vi "Main_FPGA.vi"() -> ()   [LabVIEW 2021]
uses:
  <vilib>/Platform/TimedLoop/XDataNode/timing_clust.ctl
  <vilib>/Platform/TimedLoop/XDataNode/nitl_modes.ctl
  <vilib>/Platform/TimedLoop/XDataNode/wakeup.ctl
  <vilib>/rvi/Emulation/niFpgaGetClockAttributes.vi
  <vilib>/rvi/Emulation/niFpgaSctlEmulationGetInTimedLoop.vi
  <vilib>/rvi/Emulation/niFpgaEmulationReportErrorSimple.vi
  <vilib>/rvi/Emulation/niFpgaProcessEmulError.vi
  <vilib>/rvi/Emulation/niFpgaCriticalErrorInLSC.vi
  <vilib>/rvi/eio/common/nirviEmuTemplateMethod_errors.vi
  <vilib>/Platform/TimedLoop/XDataNode/XDataNode.xnode
  <vilib>/eio/EIONode/EIONode.xnode
  <vilib>/Platform/TimedLoop/XDataNode/XDNodeRunTimeDep.lvlib
panel:
  out "CH1 SS Time (200ns)":u32
  out "CH1 Stoping":bool
  out "CH1 3rd harmonic (kHz)":fxp<+,20,10> caption="Actual frequency (kHz)" format="%#.3f"
  in  "CH2":bool
  in  "CH1":bool caption="Hardware trigger\nin enable"
  in  "Output trigger \nfrequency (Hz)":u32=30 caption="Camera frequency (Hz)" min=1 max=200
  out "CH2 Trigger Tab":enum32{"Page 1", "Page 2"}(tab) caption="CH2 trigger"
  in  "CH2 trigger":bool
  out "CH2 trigger 2":bool=TRUE
  out "Ch1 Trigger Tab":enum32{"Page 1", "Page 2"}(tab) caption="CH1 trigger"
  in  "CH1 trigger":bool
  out "CH1 trigger 2":bool=TRUE
  out "Syn tab":enum32{"Page 1", "Page 2"}(tab) caption="Synchronous trigger"
  in  "Synchronous trigger 2":bool
  out "Syn Boolean 2":bool=TRUE
  out "CH2 cooling":bool
  out "CH2 Status":T1(tab) caption="Status:"
  out "CH1 cooling":bool
  out "CH1 Status":T1(tab) caption="Status:"
  in  "Tab Control 2":enum32{"Notes", "Others"}(tab)
  out "CH2 no cooling":u32
  out "CH2 delay (200ns)":u32
  out "CH2 pulse period (200ns)":u32
  out "CH2 ON":bool
  out "CH2 Total time (200ns)":u32
  out "CH2 On time (200ns)":u32
  out "CH2 duty ratio":u32
  out "CH2 step (Hz)":u32
  out "CH2 actual f (kHz)":fxp<+,20,10> caption="Board frequency (kHz)"
  in  "CH2 maximum absolute amp":fxp<+,32,1>=0.125 caption="Maximum duty ratio"
  out "CH2 T is longer than 14 mins":bool
  out "CH2 Total T1 is longer than 4s":bool
  in  "Tab Control 1":enum32{"Notes", "Others"}(tab)
  out "CH1 step (Hz)":u32
  out "CH1 duty ratio":u32
  out "CH1 on time (200ns)":u32
  out "CH1 Pulse period (200ns)":u32
  out "CH1 ON":bool
  out "N of 5MHz":i32
  out "CH1 Total time (200ns)":u32
  out "CH1 delay (200ns)":u32
  out "CH1 no cooling":u32
  in  "CH1 maximum absolute amp":fxp<+,32,1>=0.0400000000372529 caption="Maximum duty ratio"
  out "CH1 T too long":bool
  out "CH1 T1 too long":bool
  out "DIO0":bool
  out "CH1 actual f (kHz)":fxp<+,20,10> caption="Board frequency (kHz)" format="%#.3g"
  out "CH1 Starting":bool
  in  "CH1 SS slope":u32=3 caption="Slope (duty raio% / 10ms)" max=50
  out "CH1 soft SS?":bool
  out "CH1 SS time (sec)":fxp<+,16,0>=0.0009765625 caption="Soft start/stop time (s)" format="%#.4f"
  out "CH2 elapsed time (sec)":fxp<+,40,20> caption="Elapsed time (s)" format="%#.3f"
  out "CH2 status":bool=TRUE caption="Status"
  out "CH2 3rd harmonic (kHz)":fxp<+,20,10> caption="Actual frequency (kHz)" format="%#.3f"
  in  "CH2 frequency (kHz)":fxp<+,32,20>=543.0 caption="Frequency (kHz)" format="%#.1f"
  in  "CH2 T1 time (sec)":fxp<+,16,3>=0.0009765625 caption="T1 (s)" format="%#.3f"
  in  "CH2 T2 time (sec)":fxp<+,20,10>=0.0009765625 caption="T2 (s)" format="%#.3f"
  in  "CH2 normalized amp %":u8(slide)=62 caption="Normalized amp %" max=100 scale=0.0..100.0
  out "CH2 actual amp":fxp<+,32,7> caption="Duty ratio"
  in  "CH2 delay (sec)":fxp<+,20,10>=1.0 caption="Delay (s)" format="%#.3f"
  in  "Number of CH2 pulses":u8=1 caption="Pulses #" min=1 max=25
  out "CH2 Total time (sec)":fxp<+,32,20> caption="Total time (s)" format="%#.3f"
  out "CH2 cooling time (sec)":fxp<+,44,24>=3600.0 caption="Cooling time (s)" format="%#.3f"
  out "CH1 cooling time (sec)":fxp<+,44,24>=3600.0 caption="Cooling time (s)" format="%#.3f"
  out "CH1 Total time (sec)":fxp<+,32,20> caption="Total time (s)" format="%#.3f"
  out "CH1 status":bool=TRUE caption="Status"
  in  "CH1 delay (sec)":fxp<+,20,10>=1.0 caption="Delay (s)" format="%#.3f"
  in  "Number of CH1 pulses":u8=1 caption="Pulse #" min=1 max=25
  out "CH1 actual amp":fxp<+,32,7> caption="Duty ratio"
  in  "CH1 normalized amp %":u8(slide)=59 caption="Normalized amp %" max=100 scale=0.0..100.0
  in  "System on/off":bool
  out "CH1 elapsed time (sec)":fxp<+,40,20> caption="Elapsed time (s)" format="%#.3f"
  in  "CH1 T2 time (sec)":fxp<+,20,10>=0.0009765625 caption="T2 (s)" format="%#.3f"
  in  "CH1 T1 time (sec)":fxp<+,16,3>=0.0009765625 caption="T1 (s)" format="%#.3f"
  in  "CH1 frequency (kHz)":fxp<+,32,20>=48.89990234375 caption="Frequency (kHz)" format="%#.2f"
  # "! TURN ON !\n! CIRCULATION !\n! PUMP/CHILLER !"
  # "Channel 1: ~50kHz"
  # "Trigger"
  # "%"
  # "%"
  # "Channel 2: ~550kHz"
  # "Trigger"
  # "%"
  # "%"
  # "Idle"
  # "Running"
  # "Cooling"
  # "Error: \nTotal T1 is longer than 4 s"
  # "Error: \nTotal time is longer than 14 minutes"
  # "Idle"
  # "Running"
  # "Cooling"
  # "Error: \nTotal T1 is longer than 4 s"
  # "Error: \nTotal time is longer than 14 minutes"
  # "Notes\n\n1. 12% duty ratio is about 260A, which can produce about 12.5mT field.\n\n2. The total T1 cannot be longer than 4 seconds. After running, the system must wait 50 times of total T1 to cooling down.\n\n3. The total time = Delay time + Number of pulses * (T1+T2)+Cooling time, which cannot be longer than 14 minutes."
  # "Notes\n\n1. 4.1% duty ratio is about 1000A, which can produce about 90mT field.\n\n2. The total T1 cannot be longer than 4 seconds. After running, the system must wait 50 times of total T1 to cooling down.\n\n3. The total time = Delay time + Number of pulses * (T1+T2)+Cooling time, which cannot be longer than 14 minutes."
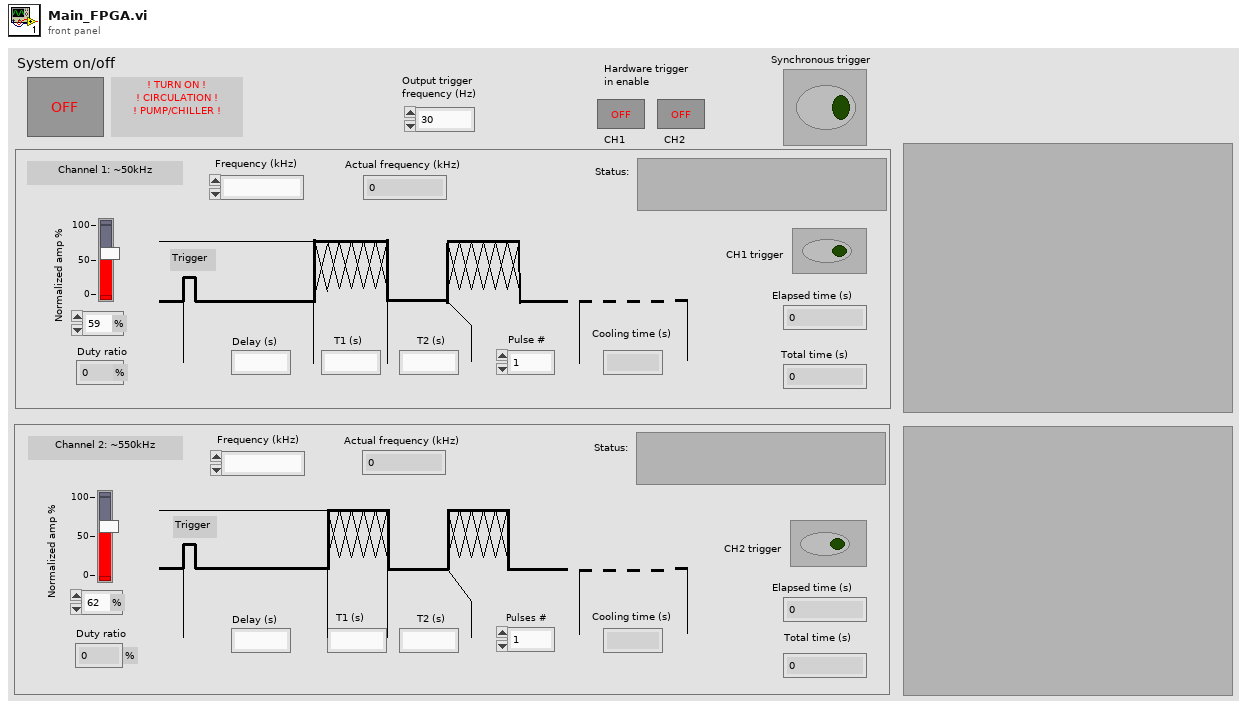
[diagram p1: front panel]
types:
  T1 = enum32{"Page 1", "Page 2", "Page 3", "Page 4", "Page 5"}
  T2 = typedef "XDNodeRunTimeDep.lvlib/timing_clust.ctl" = cluster{"Expected End [f-1]":u64, "Actual End [f-1]":u64, "Finished Late? [f-1]":bool, "Expected End [i-1]":u64, "Actual End [i-1]":u64, "Finished Late? [i-1]":bool, "Expected Start [i]":u64, "Actual Start [i]":u64, "Expected Start [f]":u64, "Actual Start [f]":u64, "Source Name":string, "Structure Name":string, "Period":i64, "Deadline":i64, "Offset":i64, "Start":i64, "Priority":i32, "Timeout":i32, "Mode":T3, "Wakeup Reason":T4, "Error":errorcluster, "Source Type":string, "Secondary Source Type":string, "Global End Time":u64, "Global Start Time":u64, "Frame Duration":u64, "Iteration Duration":u64, "Assigned CPU":i32, "I/O Scan Engine Mode":u32}
  T3 = typedef "XDNodeRunTimeDep.lvlib/nitl_modes.ctl" = enum32{"No Change", "Process missed periods, maintain original phase", "Discard missed periods, maintain original phase", "Process missed periods, ignore original phase", "Discard missed periods, ignore original phase"}
  T4 = typedef "XDNodeRunTimeDep.lvlib/wakeup.ctl" = enum32{"Normal", "Aborted", "Asynchronous wakeup", "Timing source error", "Timed loop error", "Timeout"}
  T5 = cluster{bool, bool, bool, bool, bool, bool, bool, bool}
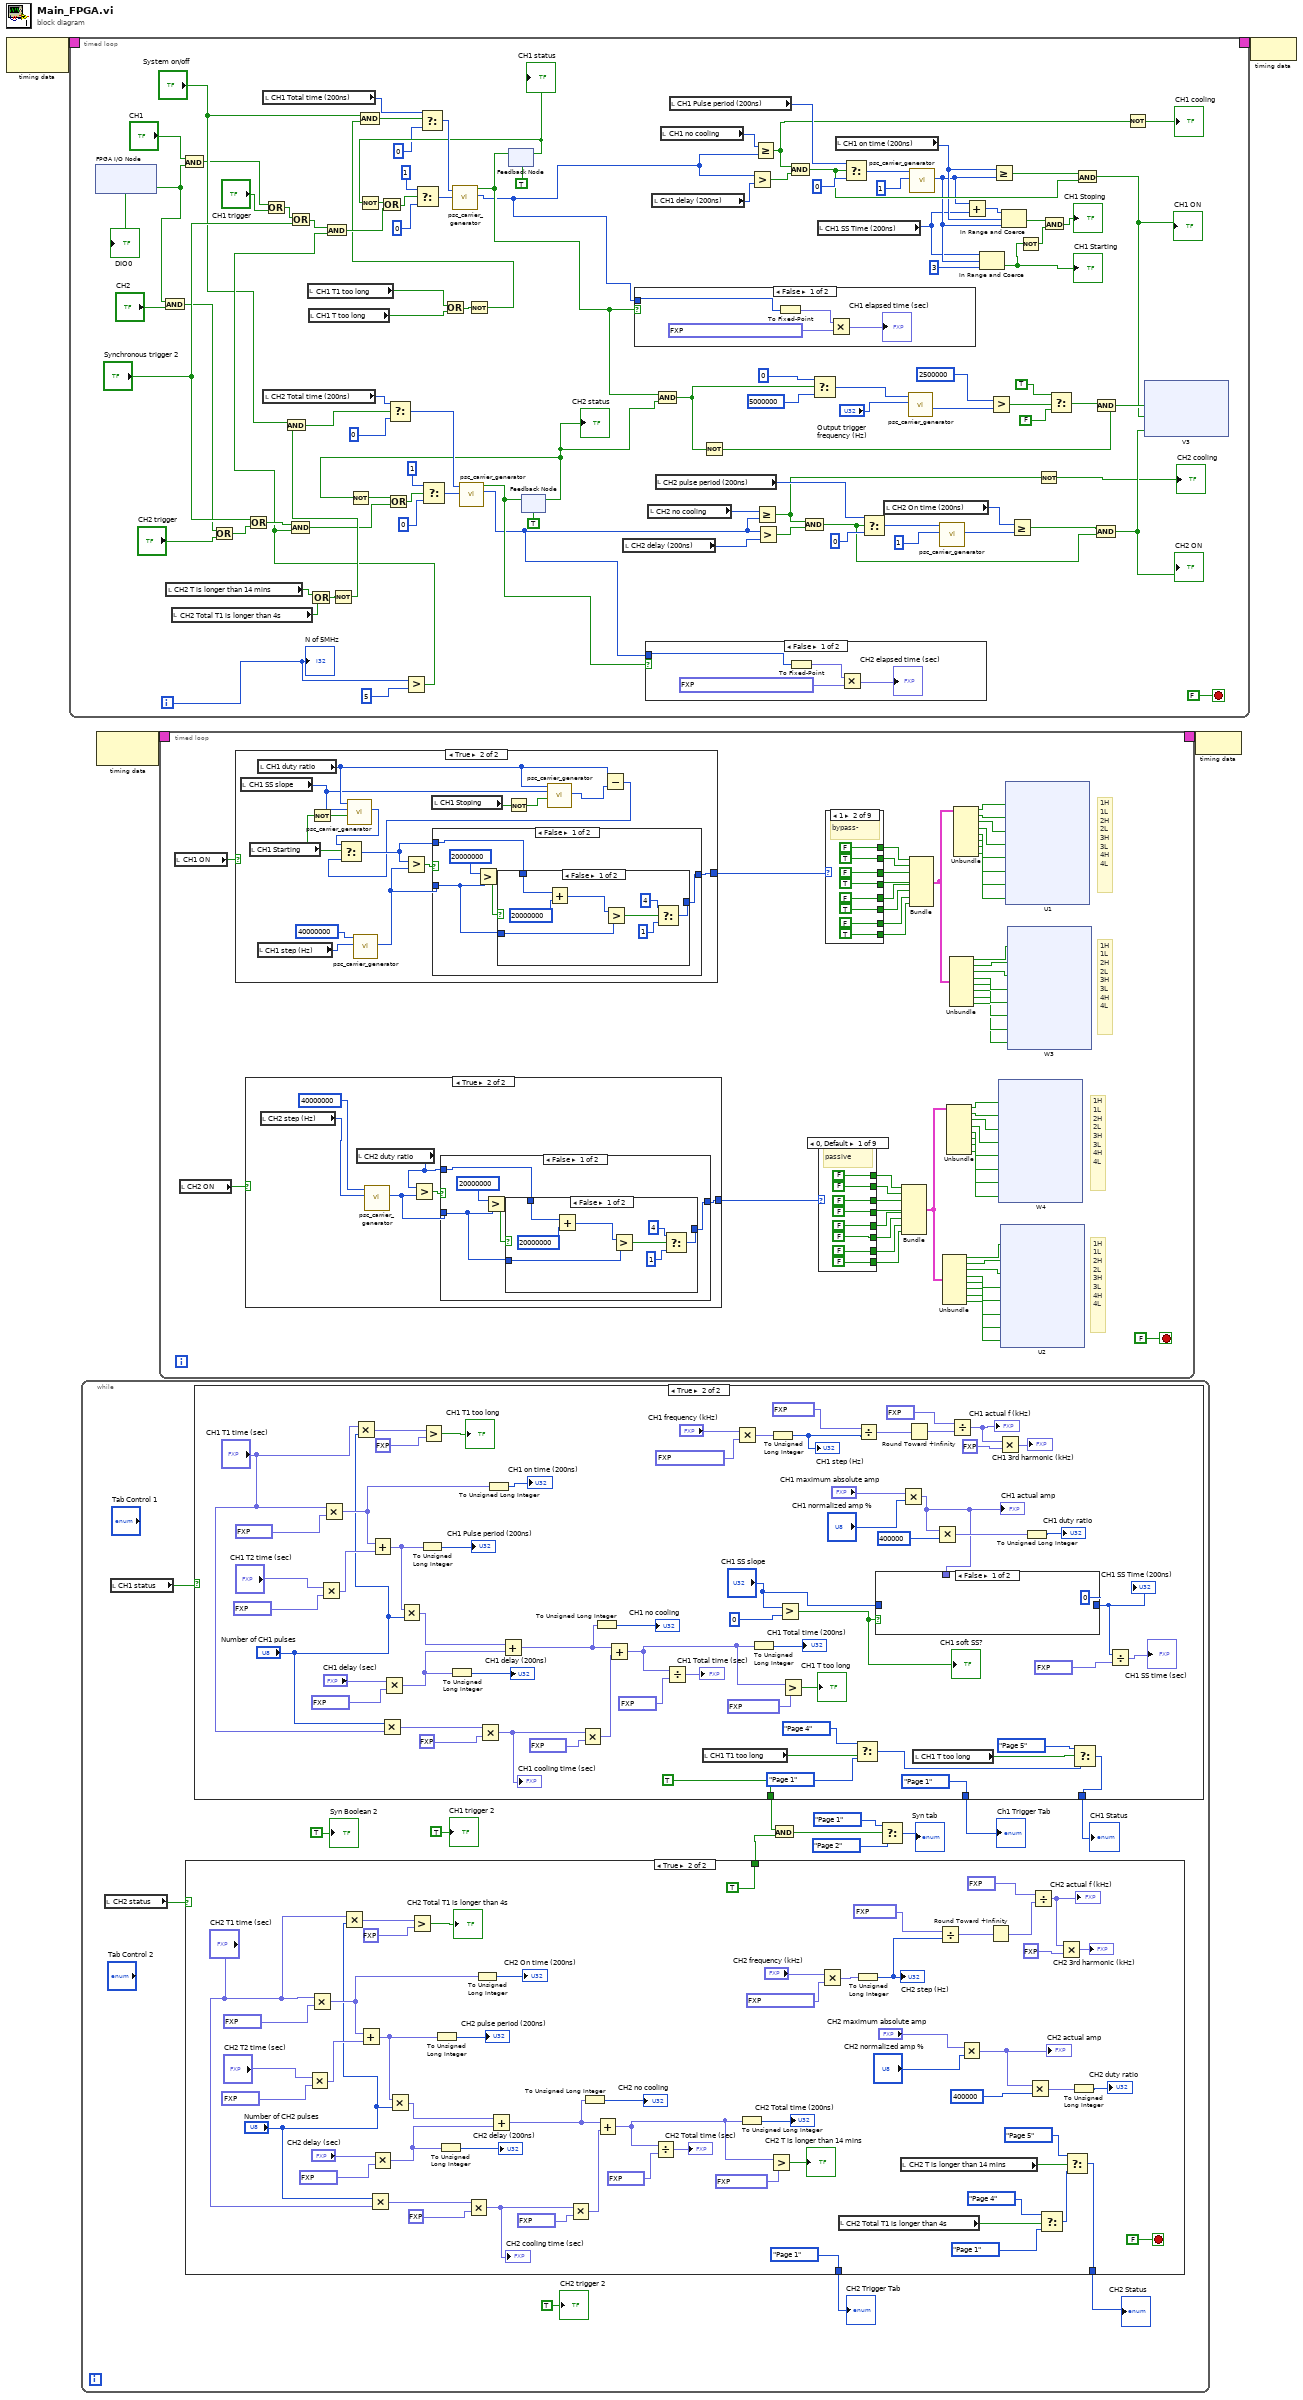
[diagram p0: block diagram]
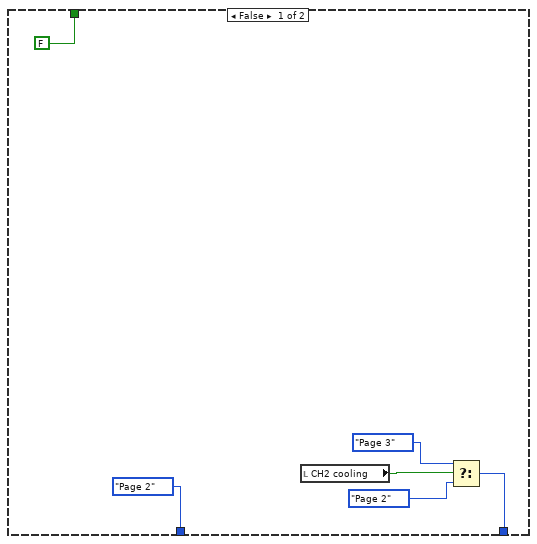
[diagram p4: hidden frame]
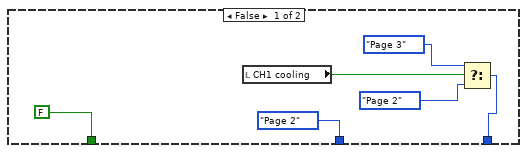
[diagram p5: hidden frame]
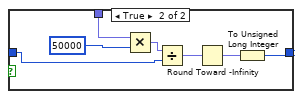
[diagram p6: hidden frame]
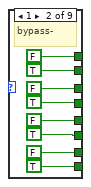
[diagram p7: hidden frame]
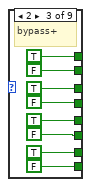
[diagram p8: hidden frame]
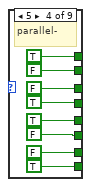
[diagram p9: hidden frame]
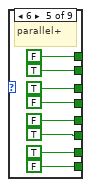
[diagram p10: hidden frame]
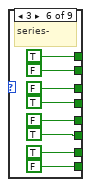
[diagram p11: hidden frame]
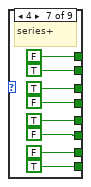
[diagram p12: hidden frame]
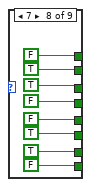
[diagram p13: hidden frame]
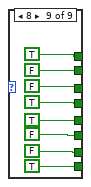
[diagram p14: hidden frame]
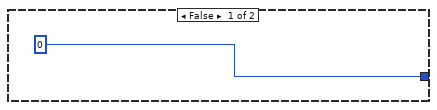
[diagram p15: hidden frame]
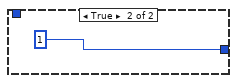
[diagram p16: hidden frame]
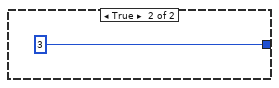
[diagram p17: hidden frame]
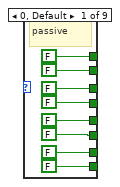
[diagram p18: hidden frame]
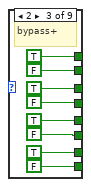
[diagram p19: hidden frame]
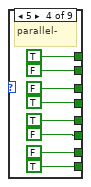
[diagram p20: hidden frame]
diagram:
  n1 = node-c288() -> (w2:T2)  [unwired: 1 in]
  n2 = timed-loop {
    timing: w2 -> [_]
    timing-out: [_] -> w1
    i -> [w85]
    stop <- FALSE stop-if-true
    n3 = xnode "FPGA I/O Node"() -> ("DIO0"=w40:bool)  [unwired: 1 in, 1 out]
    "DIO0" <- w40
    n4 = And(x=w40, y="CH2") -> (x .and. y?=w54:bool)
    n5 = local read "CH2 T is longer than 14 mins"() -> (w77:bool)
    n6 = local read "CH2 Total T1 is longer than 4s"() -> (w76:bool)
    n7 = And(x="CH1", y=w40) -> (x .and. y?=w60:bool)
    n8 = Or(x=w54, y="CH2 trigger") -> (x .or. y?=w57:bool)
    n9 = Or(x="Synchronous trigger 2", y=w57) -> (x .or. y?=w83:bool)
    n10 = local read "CH1 Total time (200ns)"() -> (w71:u32)
    n11 = local read "CH2 Total time (200ns)"() -> (w68:u32)
    n12 = Or(x=w60, y="CH1 trigger") -> (x .or. y?=w58:bool)
    n13 = Or(x=w58, y="Synchronous trigger 2") -> (x .or. y?=w82:bool)
    n14 = local read "CH1 T1 too long"() -> (w79:bool)
    n15 = local read "CH1 T too long"() -> (w78:bool)
    n16 = Or(x=w77, y=w76) -> (x .or. y?=w75:bool)
    n17 = Not(x=w75) -> (.not. x?=w96:bool)
    n18 = And(x="System on/off", y=w96) -> (x .and. y?=w63:bool)
    n19 = Select(t=w68, s=w63, f=u32 0 ("t")) -> (s? t:f=w87:u32)
    n20 = Greater?(x=w85, y=5) -> (0:w81:bool)
    n21 = And(x=w83, y=w81) -> (x .and. y?=w64:bool)
    n22 = And(x=w82, y=w81) -> (x .and. y?=w67:bool)
    n23 = Or(x=w79, y=w78) -> (x .or. y?=w80:bool)
    n24 = Not(x=w80) -> (.not. x?=w65:bool)
    n25 = And(x="System on/off", y=w65) -> (x .and. y?=w66:bool)
    n26 = Select(t=w71, s=w66, f=u32 0 ("t")) -> (s? t:f=w98:u32)
    n27 = feedback #1(TRUE ("RST_out")) -> (w74:bool)
    "CH1 status" <- w74
    n28 = Not(x=w74) -> (.not. x?=w100:bool)
    n29 = Or(x=w100, y=w67) -> (x .or. y?=w101:bool)
    n30 = Select(t=u32 1, s=w101, f=u32 0) -> (s? t:f=w103:u32)
    n31 = call "psc_carrier_generator.vi"("Step"=w103, "MAX"=w98) -> ("PSC out"=w38:u32, "RST_out"=w73:bool)  [unwired: 8 in]
    n32 = feedback-in #1(w73) -> ()
    n33 = feedback #2(TRUE ("RST_out")) -> (w72:bool)
    "CH2 status" <- w72
    n34 = Not(x=w72) -> (.not. x?=w90:bool)
    n35 = Or(x=w90, y=w64) -> (x .or. y?=w91:bool)
    n36 = Select(t=u32 1, s=w91, f=u32 0) -> (s? t:f=w93:u32)
    n37 = call "psc_carrier_generator.vi"("Step"=w93, "MAX"=w87) -> ("PSC out"=w29:u32, "RST_out"=w88:bool)  [unwired: 8 in]
    n38 = feedback-in #2(w88) -> ()
    n39 = local read "CH2 delay (200ns)"() -> (w95:u32)
    n40 = case shown="False" w73 {
      tunnel: w38 -> [w110 _]
      frame False {
        n41 = To Fixed-Point(number=w110) -> (fixed-point=w113:fxp<+,32,32>)  [unwired: 1 in]
        n42 = Multiply(x=w113, y=fxp<+,40,10> 2.0023435354232788e-07) -> (x*y=→"CH1 elapsed time (sec)":fxp<+,64,42>)
      }
      frame True {
      }
    }
    n43 = case shown="False" w88 {
      tunnel: w29 -> [w106 _]
      frame False {
        n44 = To Fixed-Point(number=w106) -> (fixed-point=w109:fxp<+,32,32>)  [unwired: 1 in]
        n45 = Multiply(x=w109, y=fxp<+,40,10> 2.0023435354232788e-07) -> (x*y=→"CH2 elapsed time (sec)":fxp<+,64,42>)
      }
      frame True {
      }
    }
    n46 = local read "CH2 no cooling"() -> (w30:u32)
    n47 = local read "CH1 delay (200ns)"() -> (w105:u32)
    n48 = And(x=w73, y=w72) -> (x .and. y?=w45:bool)
    n49 = local read "CH2 pulse period (200ns)"() -> (w21:u32)
    n50 = local read "CH1 no cooling"() -> (w39:u32)
    n51 = local read "CH1 Pulse period (200ns)"() -> (w36:u32)
    n52 = Not(x=w45) -> (.not. x?=w44:bool)
    n53 = Greater?(x=w38, y=w105) -> (0:w37:bool)
    n54 = Greater Or Equal?(x=w39, y=w38) -> (x >= y?=w17:bool)
    n55 = Greater Or Equal?(x=w30, y=w29) -> (x >= y?=w15:bool)
    n56 = Greater?(x=w29, y=w95) -> (0:w28:bool)
    n57 = And(x=w17, y=w37) -> (x .and. y?=w32:bool)
    n58 = And(x=w15, y=w28) -> (x .and. y?=w22:bool)
    n59 = Select(t=u32 0, s=w45, f=u32 5000000 ("MAX")) -> (s? t:f=w42:u32)
    n60 = local read "CH1 SS Time (200ns)"() -> (w6:u32)
    n61 = local read "CH1 on time (200ns)"() -> (w12:u32)
    n62 = Select(t=w36, s=w32, f=u32 0) -> (s? t:f=w34:u32)
    n63 = Select(t=w21, s=w22, f=u32 0) -> (s? t:f=w26:u32)
    n64 = local read "CH2 On time (200ns)"() -> (w20:u32)
    n65 = call "psc_carrier_generator.vi"("Step"="Output trigger \nfrequency (Hz)", "MAX"=w42) -> ("PSC out"=w53:u32)  [unwired: 8 in, 1 out]
    n66 = call "psc_carrier_generator.vi"("Step"=u32 1, "MAX"=w34) -> ("PSC out"=w7:u32)  [unwired: 8 in, 1 out]
    n67 = call "psc_carrier_generator.vi"("Step"=u32 1, "MAX"=w26) -> ("PSC out"=w24:u32)  [unwired: 8 in, 1 out]
    n68 = Add(x=w7, y=w6) -> (x+y=w13:u32)
    n69 = In Range and Coerce(upper limit=w6, x=w7, lower limit=u32 3) -> (In Range?=w8:bool)  [unwired: 1 out]
    "CH1 Starting" <- w8
    n70 = Greater?(x=u32 2500000 ("MAX"), y=w53) -> (0:w51:bool)
    n71 = Greater Or Equal?(x=w12, y=w7) -> (x >= y?=w14:bool)
    n72 = In Range and Coerce(upper limit=w13, x=w12, lower limit=w7) -> (In Range?=w10:bool)  [unwired: 1 out]
    n73 = Greater Or Equal?(x=w20, y=w24) -> (x >= y?=w23:bool)
    n74 = Not(x=w8) -> (.not. x?=w9:bool)
    n75 = Not(x=w15) -> (.not. x?=→"CH2 cooling":bool)
    n76 = And(x=w10, y=w9) -> (x .and. y?=→"CH1 Stoping":bool)
    n77 = Select(t=TRUE, s=w51, f=FALSE) -> (s? t:f=w47:bool)
    n78 = And(x=w14, y=w32) -> (x .and. y?=w31:bool)
    "CH1 ON" <- w31
    n79 = And(x=w23, y=w22) -> (x .and. y?=w19:bool)
    "CH2 ON" <- w19
    n80 = And(x=w47, y=w44) -> (x .and. y?=w46:bool)
    n81 = Not(x=w17) -> (.not. x?=→"CH1 cooling":bool)
    n82 = xnode "V3"("RMC/DIO39"=w46, "RMC/DIO38"=w31, "RMC/DIO6"=w19) -> ()  [unwired: 3 in, 3 out]
    "N of 5MHz" <- w85
  }
  n83 = while {
    stop <- FALSE stop-if-true
    n84 = local read "CH2 status"() -> (w130:bool)
    n85 = local read "CH1 status"() -> (w129:bool)
    n86 = case shown="True" w130 {
      tunnel: [w134 w140] -> w127
      tunnel: [FALSE TRUE] -> w121
      tunnel: [enum32{"Page 1", "Page 2"}."Page 2" ("CH2 Tab") enum32{"Page 1", "Page 2"}."Page 1" ("CH2 Tab")] -> w116
      frame False {
        n87 = local read "CH2 cooling"() -> (w137:bool)
        n88 = Select(t=T1."Page 3" ("CH1 Status"), s=w137, f=T1."Page 2" ("CH1 Status")) -> (s? t:f=w134:T1)
      }
      frame True {
        n89 = Multiply(x="CH2 T2 time (sec)", y=fxp<+,17,23> 5000000.0) -> (x*y=w172:fxp<+,37,33>)
        n90 = Multiply(x="CH2 T1 time (sec)", y=fxp<+,17,23> 5000000.0) -> (x*y=w173:fxp<+,33,26>)
        n91 = Multiply(x="CH2 T1 time (sec)", y="Number of CH2 pulses") -> (x*y=w183:fxp<+,24,11>)
        n92 = Add(x=w173, y=w172) -> (x+y=w180:fxp<+,40,33>)
        n93 = Multiply(x="Number of CH2 pulses", y="CH2 T1 time (sec)") -> (x*y=w151:fxp<+,24,11>)
        n94 = Multiply(x="CH2 delay (sec)", y=fxp<+,17,23> 5000000.0) -> (x*y=w185:fxp<+,37,33>)
        n95 = Multiply(x=w180, y="Number of CH2 pulses") -> (x*y=w181:fxp<+,48,41>)
        n96 = Greater?(x=w183, y=fxp<+,1,3> 4.0) -> (0:→"CH2 Total T1 is longer than 4s":bool)
        n97 = To Unsigned Long Integer(number=w180) -> (unsigned 32bit integer=→"CH2 pulse period (200ns)":u32)
        n98 = To Unsigned Long Integer(number=w185) -> (unsigned 32bit integer=→"CH2 delay (200ns)":u32)
        n99 = Multiply(x=w151, y=fxp<+,5,6> 50.0) -> (x*y=w191:fxp<+,29,17>)
        "CH2 cooling time (sec)" <- w191
        n100 = To Unsigned Long Integer(number=w173) -> (unsigned 32bit integer=→"CH2 On time (200ns)":u32)
        n101 = Add(x=w181, y=w185) -> (x+y=w194:fxp<+,48,41>)
        n102 = Multiply(x=w191, y=fxp<+,17,23> 5000000.0) -> (x*y=w192:fxp<+,45,39>)
        n103 = To Unsigned Long Integer(number=w194) -> (unsigned 32bit integer=→"CH2 no cooling":u32)
        n104 = Add(x=w194, y=w192) -> (x+y=w167:fxp<+,48,41>)
        n105 = Divide(x=w167, y=fxp<+,17,23> 5000000.0) -> (x/y=→"CH2 Total time (sec)":fxp<+,49,19>)
        n106 = To Unsigned Long Integer(number=w167) -> (unsigned 32bit integer=→"CH2 Total time (200ns)":u32)
        n107 = Greater?(x=w167, y=fxp<+,32,32> 4294967295.0) -> (0:→"CH2 T is longer than 14 mins":bool)
        n108 = Multiply(x="CH2 frequency (kHz)", y=fxp<+,20,9> 333.3330078125) -> (x*y=w169:fxp<+,52,29>)
        n109 = local read "CH2 Total T1 is longer than 4s"() -> (w144:bool)
        n110 = To Unsigned Long Integer(number=w169) -> (unsigned 32bit integer=w150:u32)
        "CH2 step (Hz)" <- w150
        n111 = local read "CH2 T is longer than 14 mins"() -> (w146:bool)
        n112 = Divide(x=fxp<+,17,26> 40000000.0, y=w150) -> (x/y=w189:fxp<+,49,26>)
        n113 = Multiply(x="CH2 maximum absolute amp", y="CH2 normalized amp %") -> (x*y=w177:fxp<+,40,9>)
        "CH2 actual amp" <- w177
        n114 = Round Toward +Infinity(x=w189) -> (ceil(x): smallest int >= x=w190:fxp<+,26,26>)
        n115 = Multiply(x=w177, y=u32 400000) -> (x*y=w170:fxp<+,64,41>)
        n116 = Divide(x=fxp<+,10,16> 40000.0, y=w190) -> (x/y=w149:fxp<+,36,16>)
        "CH2 actual f (kHz)" <- w149
        n117 = Select(t=T1."Page 4" ("CH1 Status"), s=w144, f=T1."Page 1" ("CH1 Status")) -> (s? t:f=w145:T1)
        n118 = Multiply(x=w149, y=fxp<+,43,26> 3.0) -> (x*y=→"CH2 3rd harmonic (kHz)":fxp<+,64,41>)
        n119 = Select(t=T1."Page 5" ("CH1 Status"), s=w146, f=w145) -> (s? t:f=w140:T1)
        n120 = To Unsigned Long Integer(number=w170) -> (unsigned 32bit integer=→"CH2 duty ratio":u32)
      }
    }
    "CH2 Status" <- w127
    "CH2 Trigger Tab" <- w116
    n121 = case shown="True" w129 {
      tunnel: [w197 w215] -> w128
      tunnel: [enum32{"Page 1", "Page 2"}."Page 2" ("Ch1 Trigger Tab") enum32{"Page 1", "Page 2"}."Page 1" ("Ch1 Trigger Tab")] -> w126
      tunnel: [FALSE TRUE] -> w122
      frame False {
        n122 = local read "CH1 cooling"() -> (w200:bool)
        n123 = Select(t=T1."Page 3" ("CH1 Status"), s=w200, f=T1."Page 2" ("CH1 Status")) -> (s? t:f=w197:T1)
      }
      frame True {
        n124 = Multiply(x="CH1 T2 time (sec)", y=fxp<+,17,23> 5000000.0) -> (x*y=w241:fxp<+,37,33>)
        n125 = Multiply(x="CH1 T1 time (sec)", y=fxp<+,17,23> 5000000.0) -> (x*y=w242:fxp<+,33,26>)
        n126 = Multiply(x="CH1 T1 time (sec)", y="Number of CH1 pulses") -> (x*y=w251:fxp<+,24,11>)
        n127 = Add(x=w242, y=w241) -> (x+y=w248:fxp<+,40,33>)
        n128 = Multiply(x="Number of CH1 pulses", y="CH1 T1 time (sec)") -> (x*y=w222:fxp<+,24,11>)
        n129 = Multiply(x="CH1 delay (sec)", y=fxp<+,17,23> 5000000.0) -> (x*y=w253:fxp<+,37,33>)
        n130 = Multiply(x=w248, y="Number of CH1 pulses") -> (x*y=w249:fxp<+,48,41>)
        n131 = To Unsigned Long Integer(number=w248) -> (unsigned 32bit integer=→"CH1 Pulse period (200ns)":u32)
        n132 = Greater?(x=w251, y=fxp<+,1,3> 4.0) -> (0:→"CH1 T1 too long":bool)
        n133 = To Unsigned Long Integer(number=w253) -> (unsigned 32bit integer=→"CH1 delay (200ns)":u32)
        n134 = Multiply(x=w222, y=fxp<+,5,6> 50.0) -> (x*y=w260:fxp<+,29,17>)
        "CH1 cooling time (sec)" <- w260
        n135 = To Unsigned Long Integer(number=w242) -> (unsigned 32bit integer=→"CH1 on time (200ns)":u32)
        n136 = Add(x=w249, y=w253) -> (x+y=w263:fxp<+,48,41>)
        n137 = Multiply(x=w260, y=fxp<+,17,23> 5000000.0) -> (x*y=w261:fxp<+,45,39>)
        n138 = To Unsigned Long Integer(number=w263) -> (unsigned 32bit integer=→"CH1 no cooling":u32)
        n139 = Add(x=w263, y=w261) -> (x+y=w236:fxp<+,48,41>)
        n140 = Divide(x=w236, y=fxp<+,17,23> 5000000.0) -> (x/y=→"CH1 Total time (sec)":fxp<+,49,19>)
        n141 = local read "CH1 T1 too long"() -> (w219:bool)
        n142 = Multiply(x="CH1 frequency (kHz)", y=fxp<+,20,9> 333.3330078125) -> (x*y=w238:fxp<+,52,29>)
        n143 = To Unsigned Long Integer(number=w236) -> (unsigned 32bit integer=→"CH1 Total time (200ns)":u32)
        n144 = To Unsigned Long Integer(number=w238) -> (unsigned 32bit integer=w257:u32)
        "CH1 step (Hz)" <- w257
        n145 = Greater?(x="CH1 SS slope", y=u32 0) -> (0:w207:bool)
        "CH1 soft SS?" <- w207
        n146 = Greater?(x=w236, y=fxp<+,32,32> 4294967295.0) -> (0:→"CH1 T too long":bool)
        n147 = Select(t=T1."Page 4" ("CH1 Status"), s=w219, f=T1."Page 1" ("CH1 Status")) -> (s? t:f=w220:T1)
        n148 = Divide(x=fxp<+,17,26> 40000000.0, y=w257) -> (x/y=w258:fxp<+,49,26>)
        n149 = Multiply(x="CH1 maximum absolute amp", y="CH1 normalized amp %") -> (x*y=w205:fxp<+,40,9>)
        "CH1 actual amp" <- w205
        n150 = case shown="False" w207 {
          tunnel: w205 -> [_ w271]
          tunnel: "CH1 SS slope" -> [_ w265]
          tunnel: [u32 0 ("y") w268] -> w202
          frame False {
          }
          frame True {
            n151 = Multiply(x=w271, y=u32 50000) -> (x*y=w269:fxp<+,64,41>)
            n152 = Divide(x=w269, y=w265) -> (x/y=w267:fxp<+,64,41>)
            n153 = Round Toward -Infinity(1:w267) -> (0:w266:fxp<+,41,41>)
            n154 = To Unsigned Long Integer(number=w266) -> (unsigned 32bit integer=w268:u32)
          }
        }
        "CH1 SS Time (200ns)" <- w202
        n155 = Round Toward +Infinity(x=w258) -> (ceil(x): smallest int >= x=w259:fxp<+,26,26>)
        n156 = local read "CH1 T too long"() -> (w221:bool)
        n157 = Multiply(x=w205, y=u32 400000) -> (x*y=w239:fxp<+,64,41>)
        n158 = Divide(x=fxp<+,10,16> 40000.0, y=w259) -> (x/y=w209:fxp<+,36,16>)
        "CH1 actual f (kHz)" <- w209
        n159 = Multiply(x=w209, y=fxp<+,43,26> 3.0) -> (x*y=→"CH1 3rd harmonic (kHz)":fxp<+,64,41>)
        n160 = To Unsigned Long Integer(number=w239) -> (unsigned 32bit integer=→"CH1 duty ratio":u32)
        n161 = Select(t=T1."Page 5" ("CH1 Status"), s=w221, f=w220) -> (s? t:f=w215:T1)
        n162 = Divide(x=w202, y=fxp<+,17,23> 5000000.0) -> (x/y=→"CH1 SS time (sec)":fxp<+,33,10>)
      }
    }
    "CH1 Status" <- w128
    "Ch1 Trigger Tab" <- w126
    n163 = And(x=w122, y=w121) -> (x .and. y?=w120:bool)
    n164 = Select(t=enum32{"Page 1", "Page 2"}."Page 1" ("Ch1 Trigger Tab"), s=w120, f=enum32{"Page 1", "Page 2"}."Page 2" ("Ch1 Trigger Tab")) -> (s? t:f=→"Syn tab":enum32{"Page 1", "Page 2"})
    "Syn Boolean 2" <- TRUE ("Syn Boolean 2")
    "CH1 trigger 2" <- TRUE ("CH1 trigger 2")
    "CH2 trigger 2" <- TRUE ("CH2 trigger 2")
  }
  n165 = node-c288() -> (w4:T2)  [unwired: 1 in]
  n166 = timed-loop {
    timing: w4 -> [_]
    timing-out: [_] -> w3
    stop <- FALSE stop-if-true
    # "1H\n1L\n2H\n2L\n3H\n3L\n4H\n4L"
    # "1H\n1L\n2H\n2L\n3H\n3L\n4H\n4L"
    # "1H\n1L\n2H\n2L\n3H\n3L\n4H\n4L"
    # "1H\n1L\n2H\n2L\n3H\n3L\n4H\n4L"
    n167 = local read "CH1 ON"() -> (w302:bool)
    n168 = local read "CH2 ON"() -> (w276:bool)
    n169 = case shown="True" w302 {
      tunnel: [u8 0 ("t") w508] -> w273
      frame False {
      }
      frame True {
        n170 = local read "CH1 SS slope"() -> (w495:u32)
        n171 = local read "CH1 Starting"() -> (w497:bool)
        n172 = local read "CH1 step (Hz)"() -> (w505:u32)
        n173 = local read "CH1 duty ratio"() -> (w496:u32)
        n174 = Not(x=w497) -> (.not. x?=w498:bool)
        n175 = call "psc_carrier_generator.vi"("RST_in"=w498, "Step"=w495, "MAX"=w496) -> ("PSC out"=w494:u32)  [unwired: 7 in, 1 out]
        n176 = call "psc_carrier_generator.vi"("Step"=w505, "MAX"=u32 40000000) -> ("PSC out"=w506:u32)  [unwired: 8 in, 1 out]
        n177 = local read "CH1 Stoping"() -> (w502:bool)
        n178 = Not(x=w502) -> (.not. x?=w501:bool)
        n179 = call "psc_carrier_generator.vi"("RST_in"=w501, "Step"=w495, "MAX"=w496) -> ("PSC out"=w503:u32)  [unwired: 7 in, 1 out]
        n180 = Subtract(x=w496, y=w503) -> (x-y=w499:u32)
        n181 = Select(t=w494, s=w497, f=w499) -> (s? t:f=w500:u32)
        n182 = Greater?(x=w500, y=w506) -> (0:w507:bool)
        n183 = case shown="False" w507 {
          tunnel: [w511 u8 3 ("t")] -> w508
          tunnel: w506 -> [w510 _]
          tunnel: w500 -> [w509 _]
          frame False {
            n184 = Greater?(x=u32 20000000, y=w510) -> (0:w512:bool)
            n185 = case shown="False" w512 {
              tunnel: [w517 u8 1 ("t")] -> w511
              tunnel: w510 -> [w521 _]
              tunnel: w509 -> [w514 _]
              frame False {
                n186 = Add(x=w514, y=u32 20000000) -> (x+y=w516:u32)
                n187 = Greater?(x=w516, y=w521) -> (0:w520:bool)
                n188 = Select(t=u8 4, s=w520, f=u8 1 ("t")) -> (s? t:f=w517:u8)
              }
              frame True {
              }
            }
          }
          frame True {
          }
        }
      }
    }
    n189 = case shown="True" w276 {
      tunnel: [u8 0 ("t") w405] -> w272
      frame False {
      }
      frame True {
        n190 = local read "CH2 step (Hz)"() -> (w401:u32)
        n191 = local read "CH2 duty ratio"() -> (w403:u32)
        n192 = call "psc_carrier_generator.vi"("Step"=w401, "MAX"=u32 40000000) -> ("PSC out"=w402:u32)  [unwired: 8 in, 1 out]
        n193 = Greater?(x=w403, y=w402) -> (0:w404:bool)
        n194 = case shown="False" w404 {
          tunnel: [w408 u8 3 ("t")] -> w405
          tunnel: w402 -> [w407 _]
          tunnel: w403 -> [w406 _]
          frame False {
            n195 = Greater?(x=u32 20000000, y=w407) -> (0:w409:bool)
            n196 = case shown="False" w409 {
              tunnel: [w414 u8 1 ("t")] -> w408
              tunnel: w407 -> [w418 _]
              tunnel: w406 -> [w411 _]
              frame False {
                n197 = Add(x=w411, y=u32 20000000) -> (x+y=w413:u32)
                n198 = Greater?(x=w413, y=w418) -> (0:w417:bool)
                n199 = Select(t=u8 4, s=w417, f=u8 1 ("t")) -> (s? t:f=w414:u8)
              }
              frame True {
              }
            }
          }
          frame True {
          }
        }
      }
    }
    n200 = case shown="0, Default" w272 {
      tunnel: [FALSE TRUE FALSE FALSE TRUE FALSE TRUE TRUE FALSE] -> w300
      tunnel: [FALSE FALSE TRUE FALSE TRUE FALSE TRUE TRUE FALSE] -> w299
      tunnel: [FALSE TRUE FALSE TRUE FALSE TRUE FALSE FALSE TRUE] -> w298
      tunnel: [FALSE FALSE TRUE TRUE FALSE FALSE TRUE FALSE TRUE] -> w296
      tunnel: [FALSE TRUE FALSE FALSE TRUE TRUE FALSE TRUE FALSE] -> w295
      tunnel: [FALSE FALSE TRUE FALSE TRUE TRUE FALSE TRUE FALSE] -> w294
      tunnel: [FALSE TRUE FALSE TRUE FALSE FALSE TRUE FALSE TRUE] -> w293
      tunnel: [FALSE FALSE TRUE TRUE FALSE TRUE FALSE FALSE TRUE] -> w297
      frame 0, Default {
        # "passive"
      }
      frame 1 {
        # "bypass-"
      }
      frame 2 {
        # "bypass+"
      }
      frame 5 {
        # "parallel-"
      }
      frame 6 {
        # "parallel+"
      }
      frame 3 {
        # "series-"
      }
      frame 4 {
        # "series+"
      }
      frame 7 {
      }
      frame 8 {
      }
    }
    n201 = case shown="1" w273 {
      tunnel: [FALSE TRUE FALSE FALSE TRUE FALSE TRUE TRUE FALSE] -> w326
      tunnel: [FALSE FALSE TRUE FALSE TRUE FALSE TRUE TRUE FALSE] -> w325
      tunnel: [FALSE TRUE FALSE TRUE FALSE TRUE FALSE FALSE TRUE] -> w324
      tunnel: [FALSE FALSE TRUE TRUE FALSE FALSE TRUE FALSE TRUE] -> w322
      tunnel: [FALSE TRUE FALSE FALSE TRUE TRUE FALSE TRUE FALSE] -> w321
      tunnel: [FALSE FALSE TRUE FALSE TRUE TRUE FALSE TRUE FALSE] -> w320
      tunnel: [FALSE TRUE FALSE TRUE FALSE FALSE TRUE FALSE TRUE] -> w319
      tunnel: [FALSE FALSE TRUE TRUE FALSE TRUE FALSE FALSE TRUE] -> w323
      frame 0, Default {
        # "passive"
      }
      frame 1 {
        # "bypass-"
      }
      frame 2 {
        # "bypass+"
      }
      frame 5 {
        # "parallel-"
      }
      frame 6 {
        # "parallel+"
      }
      frame 3 {
        # "series-"
      }
      frame 4 {
        # "series+"
      }
      frame 7 {
      }
      frame 8 {
      }
    }
    n202 = Bundle(w297, w300, w299, w298, w296, w295, w294, w293) -> (w275:T5)  [unwired: 1 in]
    n203 = Bundle(w323, w326, w325, w324, w322, w321, w320, w319) -> (w274:T5)  [unwired: 1 in]
    n204 = Unbundle(w275) -> (w284:bool, w283:bool, w282:bool, w281:bool, w280:bool, w279:bool, w278:bool, w277:bool)
    n205 = Unbundle(w275) -> (w292:bool, w291:bool, w290:bool, w289:bool, w288:bool, w287:bool, w286:bool, w285:bool)
    n206 = Unbundle(w274) -> (w310:bool, w309:bool, w308:bool, w307:bool, w306:bool, w305:bool, w304:bool, w303:bool)
    n207 = Unbundle(w274) -> (w318:bool, w317:bool, w316:bool, w315:bool, w314:bool, w313:bool, w312:bool, w311:bool)
    n208 = xnode "W4"("RMC/DIO50"=w292, "RMC/DIO18"=w291, "RMC/DIO17"=w290, "RMC/DIO49"=w289, "RMC/DIO16"=w288, "RMC/DIO81"=w287, "RMC/DIO80"=w286, "RMC/DIO48"=w285) -> ()  [unwired: 8 in, 8 out]
    n209 = xnode "U2"("RMC/DIO63"=w284, "RMC/DIO95"=w283, "RMC/DIO31"=w282, "RMC/DIO62"=w281, "RMC/DIO94"=w280, "RMC/DIO30"=w279, "RMC/DIO93"=w278, "RMC/DIO61"=w277) -> ()  [unwired: 8 in, 8 out]
    n210 = xnode "U1"("RMC/DIO47"=w318, "RMC/DIO15"=w317, "RMC/DIO46"=w316, "RMC/DIO79"=w315, "RMC/DIO14"=w314, "RMC/DIO78"=w313, "RMC/DIO13"=w312, "RMC/DIO45"=w311) -> ()  [unwired: 8 in, 8 out]
    n211 = xnode "W3"("RMC/DIO2"=w310, "RMC/DIO66"=w309, "RMC/DIO1"=w308, "RMC/DIO33"=w307, "RMC/DIO65"=w306, "RMC/DIO32"=w305, "RMC/DIO0"=w304, "RMC/DIO64"=w303) -> ()  [unwired: 8 in, 8 out]
  }
  n212 = node-c288(w3) -> ()
  n213 = node-c288(w1) -> ()
